vi "AuMT8852B Operation Mode.vi"(5 "Mode (Script)":T1(ring), 7 "Set/Get (Set)":enum16{"Set", "Get"}(ring), 8 "error in (no error)":errorcluster, 11 "VISA session":refnum<visa-resource-name>) -> (0 "error out":errorcluster, 2 "error code":i32, 3 "VISA session out":refnum<visa-resource-name>, 4 "Mode out":T1(ring))   [LabVIEW 2017]
doc: "Anritsu MT8852B Bluetooth Tester\n\nWhether the instrument is in script test mode or in one of the individual tests.\n\nINPUTS\nSet/Get - whether the value is being sent to or retrieved from the instrument.\nMode - operation mode to send to the tester.\n\nOUTPUTS\nMode out - current operation mode of the tester."
uses:
  <instrlib>/aumt8852B/General/Utilities/MT8850 Attribute ID.ctl
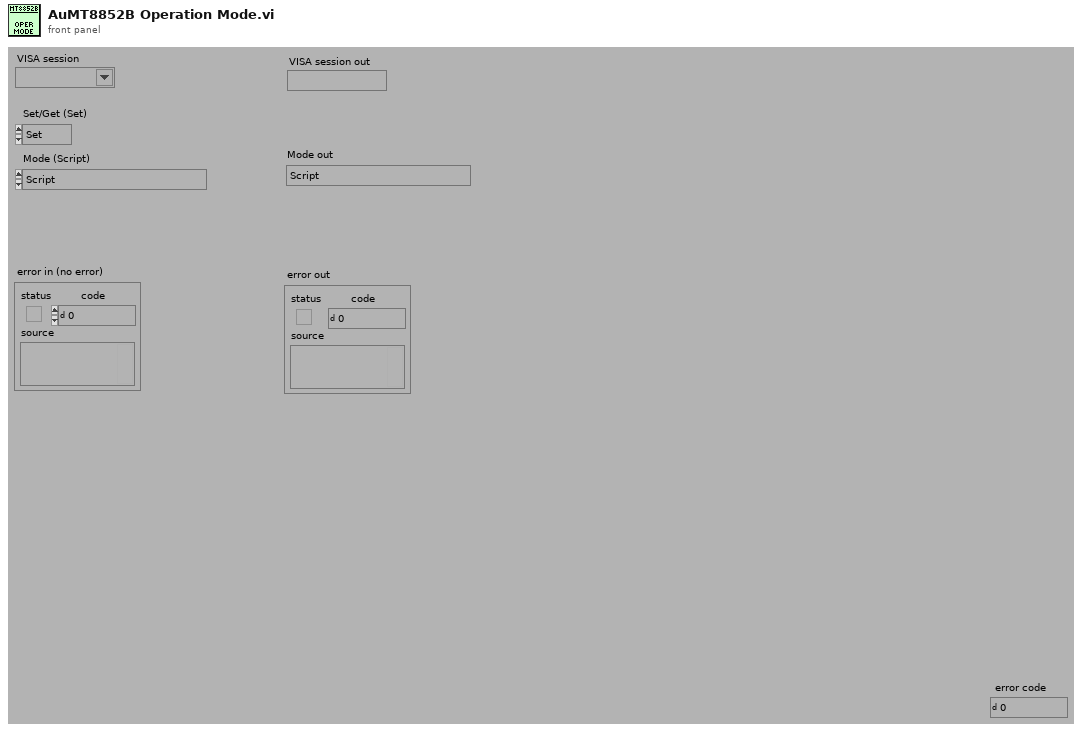
[diagram p1: front panel]
types:
  T1 = enum16{"Script", "Output power", "Power control", "Modulation characteristics", "Initial carrier", "Carrier drift", "Single slot sensitivity", "Multiple slot sensitivity", "Maximum input power", "EDR Relative transmit power", "EDR Carrier frequency and accuracy", "EDR Differential phase", "EDR Sensitivity", "EDR BER floor sensitivity", "EDR Maximum input power", "Signal generator", "EDR signal generator", "CW measurement", "EDR CW measurement"}
  T2 = typedef "MT8850 Attribute ID.ctl" = enum16{"Operation mode", "Selected script", "EUT address source", "EUT Address", "EUT HCI RS232 Baud Rate", "Tester GPIB Address", "Tester RS232 Baud Rate", "Tester Bluetooth Address", "Tester Contrast", "Tester Key Click On", "Tester Modulation Index", "Tester Poll-Null Mode", "Tester Power Range", "Tester RS232 Mode", "Beep on Illegal Entry", "Display User Text", "User Text", "Calibration TX Modulation DAC", "Calibration RX Channel", "Calibration TX Channel", "Calibration TX Power", "Calibration Use TX Table", "Inquiry Request User-friendly Name", "Inquiry Number of Responses", "Inquiry Timeout", "Script Frequency Display", "Script Loop Count", "Script Loop Continuously", "Script Loop Stop on Fail", "Link timeout", "Page timeout", "Filter bandwidth", "SCO air code", "SCO bit position", "SCO input code", "SCO input data", "SCO input sample size", "SCO loopback mode", "SCO packet type", "SCO tone generator", "Tester page scan repetition mode", "Tester follow test mode", "Tester authentication state", "Tester authentication pin code", "Tester authentication pin length"}
  T3 = typedef "Attribute Status.ctl" = enum16{"No I/O needed", "I/O needed"}
  T4 = enum16{"Script", "Output power", "Power control", "Modulation characteristics", "Initial carrier", "Carrier drift", "Single slot sensitivity", "Multiple slot sensitivity", "Maximum input power", "Signal generator", "CW measurement"}[]
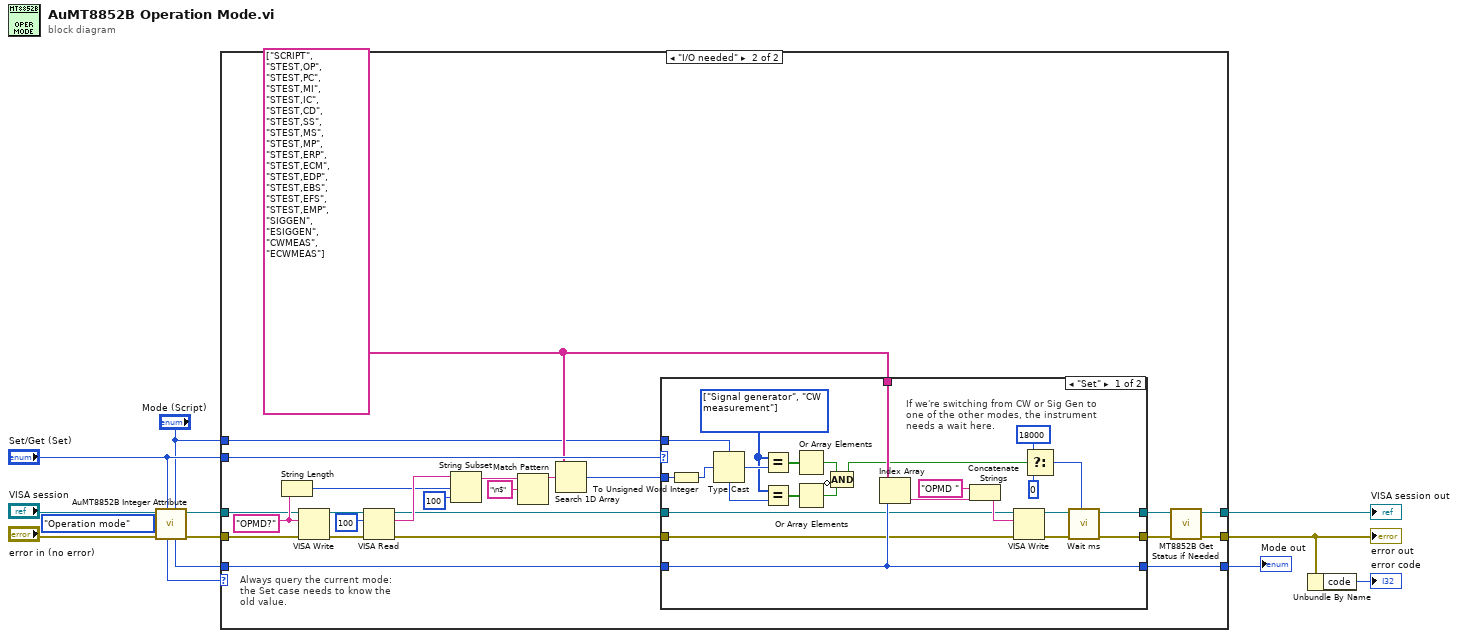
[diagram p0: block diagram]
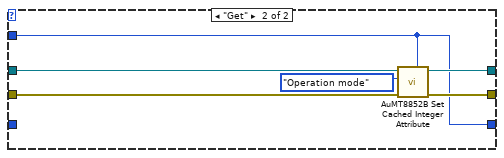
[diagram p3: hidden frame]
diagram:
  n1 = call <instrlib>:"AuMT8852B Integer Attribute.vi"("Value (0)"="Mode (Script)", "Set/Get (Set)"="Set/Get (Set)", "error in (no error)"="error in (no error)", "Attribute ID"=MT8850_Attribute_ID."Operation mode", "VISA session"="VISA session") -> ("error out"=w6:errorcluster, "VISA session out"=w7:refnum<visa-resource-name>, "Value out"=w9:i32, "Status"=w5:T3)  [unwired: 3 in]
  n2 = case shown="\"I/O needed\"" w5 {
    tunnel: "Set/Get (Set)" -> [_ w40]
    tunnel: w9 -> [w16 w39]
    tunnel: [w14 w34] -> w3
    tunnel: [w15 w35] -> w8
    tunnel: w7 -> [w15 w29]
    tunnel: w6 -> [w14 w30]
    tunnel: [w16 w38] -> w1
    tunnel: "Mode (Script)" -> [_ w19]
    frame "No I/O needed", Default {
    }
    frame "I/O needed" {
      w32 = "OPMD?" ("write buffer (\"\")")
      w20 = string[] ["SCRIPT", "STEST,OP", "STEST,PC", "STEST,MI", "STEST,IC", "STEST,CD", "STEST,SS", "STEST,MS", "STEST,MP", "STEST,ERP", "STEST,ECM", "STEST,EDP", "STEST,EBS", "STEST,EFS", "STEST,EMP", "SIGGEN", "ESIGGEN", "CWMEAS", "ECWMEAS"] ("Array Constant")
      # "Always query the current mode:\nthe Set case needs to know the\nold value."
      n3 = String Length(string=w32) -> (length=w17:i32)
      n4 = VISA Write(VISA resource name=w29, write buffer=w32, error in (no error)=w30) -> (VISA resource name out=w27:refnum<visa-resource-name>, error out=w28:errorcluster)  [unwired: 1 out]
      n5 = VISA Read(VISA resource name=w27, byte count=u32 100 ("byte count (0)"), error in (no error)=w28) -> (VISA resource name out=w22:refnum<visa-resource-name>, read buffer=w33:string, error out=w21:errorcluster)  [unwired: 1 out]
      n6 = String Subset(string=w33, offset (0)=w17, length (rest)=100 ("length (rest)")) -> (substring=w23:string)
      n7 = Match Pattern(string=w23, regular expression="\n$") -> (before substring=w31:string)  [unwired: 1 in, 3 out]
      n8 = Search 1D Array(1D array=w20, element=w31) -> (index of element=w18:i32)  [unwired: 1 in]
      n9 = case shown="\"Set\"" w40 {
        tunnel: [w46 w69] -> w36
        tunnel: w20 -> [w64 _]
        tunnel: w39 -> [w63 _]
        tunnel: [w47 w70] -> w37
        tunnel: w22 -> [w51 w66]
        tunnel: w21 -> [w50 w65]
        tunnel: [w63 w67] -> w38
        tunnel: w19 -> [w56 _]
        tunnel: w18 -> [w59 w67]
        frame "Set" {
          w55 = T4 [enum."Signal generator", enum."CW measurement"] items=["Script", "Output power", "Power control", "Modulation characteristics", "Initial carrier", "Carrier drift", "Single slot sensitivity", "Multiple slot sensitivity", "Maximum input power", "Signal generator", "CW measurement"] ("Array Constant")
          # "If we're switching from CW or Sig Gen to\none of the other modes, the instrument\nneeds a wait here."
          n10 = To Unsigned Word Integer(number=w59) -> (unsigned 16bit integer=w41:u16)
          n11 = Type Cast(type=w56, x=w41) -> (*(type *) &x=w58:T1)
          n12 = Equal?(x=w55, y=w58) -> (x = y?=w57:bool[])
          n13 = Equal?(x=w55, y=w56) -> (x = y?=w54:bool[])
          n14 = Or Array Elements(Boolean array=w57) -> (logical OR=w52:bool)
          n15 = Or Array Elements(Boolean array=w54) -> (logical OR=w53:bool)
          n16 = Compound Arithmetic op=AND(w52, invert w53) -> (w45:bool)
          n17 = Index Array(array=w64, index=w63) -> (element=w61:string)
          n18 = Concatenate Strings("OPMD " ("Substring"), w61) -> (w62:string)
          n19 = VISA Write(VISA resource name=w51, write buffer=w62, error in (no error)=w50) -> (VISA resource name out=w48:refnum<visa-resource-name>, error out=w49:errorcluster)  [unwired: 1 out]
          n20 = Select(t=u32 18000 ("Wait (1000 ms)"), s=w45, f=u32 0) -> (s? t:f=w42:u32)
          n21 = call <instrlib>:"Wait ms.vi"("Wait (1000 ms)"=w42, "error in (no error)"=w49, "VISA Session"=w48) -> ("error out"=w46:errorcluster, "VISA Session out"=w47:refnum<visa-resource-name>)  [unwired: 7 in]
        }
        frame "Get" {
          n22 = call <instrlib>:"AuMT8852B Set Cached Integer Attribute.vi"("Value (0)"=w67, "error in (no error)"=w65, "Attribute ID"=MT8850_Attribute_ID."Operation mode", "VISA session"=w66) -> ("error out"=w69:errorcluster, "VISA session out"=w70:refnum<visa-resource-name>)  [unwired: 6 in]
        }
      }
      n23 = call <instrlib>:"MT8852B Get Status if Needed.vi"("error in (no error)"=w36, "VISA session"=w37) -> ("error out"=w34:errorcluster, "VISA session out"=w35:refnum<visa-resource-name>)  [unwired: 8 in]
    }
  }
  "error out" <- w3
  "VISA session out" <- w8
  "Mode out" <- w1
  n24 = Unbundle By Name(w3) -> ("code"=→"error code":i32)
